vi "Test Worker Registered with Worker Handler after Handling Job.vi"(8 "error in (no error)":errorcluster, 11 "Worker Test in":refnum<class "Worker Test.lvclass">) -> (0 "error out":errorcluster, 3 "Worker Test out":refnum<class "Worker Test.lvclass">)   [LabVIEW 2020, in "Worker Test.lvclass"]
uses:
  Worker Test.lvclass
  C:/Program Files (x86)/National Instruments/LabVIEW 2020/vi.lib/Asteme/LUnit/Test Case.lvclass
  Mock Worker/Mock Job Handler.lvclass
  C:/Users/anton/Documents/GitHub/Triarc-Examples/Coffee Shop/Process Job/Job Handler.lvclass
  <vilib>/Asteme/Triarc Framework/Process/Process.lvclass/Process.ctl
  <vilib>/Asteme/LUnit/Test Case.lvclass/Test Case.ctl
  <vilib>/Asteme/LUnit/LUnit Assertion Result.lvclass/LUnit Assertion Result.ctl
  <vilib>/Asteme/Triarc Framework/Process/Private/SubVIs/Wait for finish.vi
  <vilib>/Asteme/Triarc Framework/Process/Protected/Messaging/Enqueue Message.vi
  <vilib>/Asteme/Triarc Framework/Process/Private/SubVIs/Set Lifecycle State.vi
  <vilib>/Asteme/Triarc Framework/Process/Public/Lifecycle/Get Lifecycle State.vi
  <vilib>/Asteme/LUnit/Palette/Pass If.vi
  <vilib>/Asteme/LUnit/Set Assertion Type.vi
  <vilib>/AdvancedString/1D String Array to Delimited String.vi
  <vilib>/Utility/error.llb/Clear Errors.vi
  <vilib>/Asteme/LUnit/Palette/Fail.vi
  <vilib>/Asteme/LUnit/Palette/Pass.vi
  <vilib>/Asteme/LUnit/LUnit Write Assertion Type.vi
  <vilib>/Asteme/LUnit/Add test result.vi
  <vilib>/Asteme/LUnit/LUnit Write Passed.vi
  <vilib>/Asteme/LUnit/LUnit Get Test Case.vi
  <vilib>/Asteme/LUnit/Assertion Result/LUnit Get Test Name.vi
  <vilib>/Asteme/LUnit/LUnit Write Message.vi
  <vilib>/Asteme/LUnit/LUnit Write Description.vi
  <vilib>/Asteme/LUnit/Read Test Case Name.vi
  Worker/Worker.lvclass
  C:/Program Files (x86)/National Instruments/LabVIEW 2020/vi.lib/Asteme/Triarc Framework/Process/Process.lvclass
  <vilib>/Utility/error.llb/Error Cluster From Error Code.vi
  <vilib>/Asteme/LUnit/LUnit Assertion Result.lvclass
  <vilib>/Asteme/Triarc Framework/Process/Process.lvclass
  <vilib>/Asteme/LUnit/Test Case.lvclass
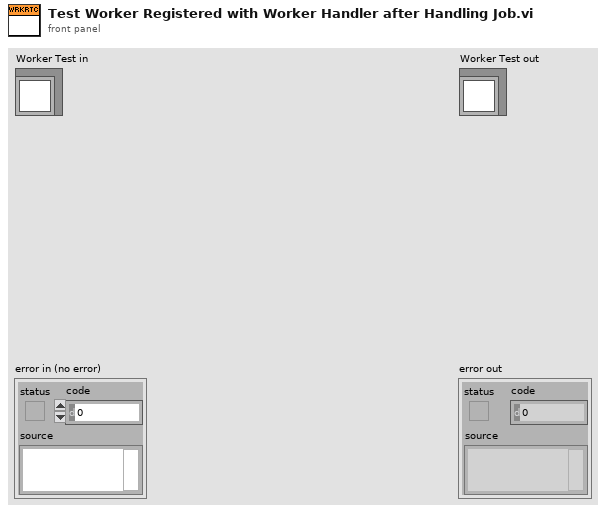
[diagram p1: front panel]
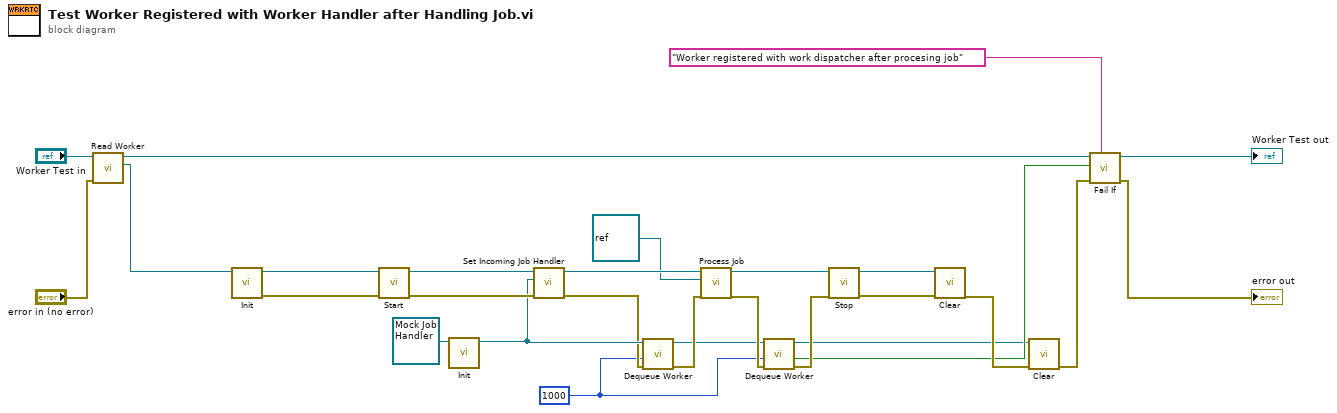
[diagram p0: block diagram]
diagram:
  w1 = 1000 ("timeout in ms (-1)")
  n1 = call "Read Worker.vi"("error in (no error)"="error in (no error)", "Worker Test in"="Worker Test in") -> ("Worker"=w23:refnum<class "Worker.lvclass">, "Worker Test out"=w25:refnum<class "Worker Test.lvclass">)  [unwired: 7 in, 1 out]
  n2 = call-dynamic "Init.vi"("View In"=w23) -> ("error out"=w22:errorcluster, "View Out"=w19:refnum<class "Worker.lvclass">)  [unwired: 9 in]
  n3 = call <vilib>:"Start.vi"("error in (no error)"=w22, "Process In"=w19) -> ("error out"=w18:errorcluster, "Process Out"=w16:refnum<class "Worker.lvclass">)  [unwired: 8 in]
  n4 = call-dynamic "Init.vi"("Mock Job Handler In"=refnum<class "Mock Job Handler.lvclass"> refnum ("Mock Worker In")) -> ("Mock Job Handler Out"=w14:refnum<class "Mock Job Handler.lvclass">)  [unwired: 9 in, 1 out]
  n5 = call "Set Incoming Job Handler.vi"("error in (no error)"=w18, "Job Handler"=w14, "Worker In"=w16) -> ("error out"=w13:errorcluster, "Worker Out"=w9:refnum<class "Worker.lvclass">)  [unwired: 7 in]
  n6 = call "Dequeue Worker.vi"("error in (no error)"=w13, "timeout in ms (-1)"=w1, "Mock Job Handler In"=w14) -> ("error out"=w12:errorcluster, "Mock Job Handler Out"=w3:refnum<class "Mock Job Handler.lvclass">)  [unwired: 5 in, 2 out]
  n7 = call-dynamic "Process Job.vi"("error in (no error)"=w12, "Job"=refnum<class> refnum ("Task"), "Worker In"=w9) -> ("error out"=w6:errorcluster, "Worker Out"=w8:refnum<class "Worker.lvclass">)  [unwired: 7 in]
  n8 = call "Dequeue Worker.vi"("error in (no error)"=w6, "timeout in ms (-1)"=w1, "Mock Job Handler In"=w3) -> ("error out"=w5:errorcluster, "timed out?"=w4:bool, "Mock Job Handler Out"=w2:refnum<class "Mock Job Handler.lvclass">)  [unwired: 5 in, 1 out]
  n9 = call <vilib>:"Stop.vi"("error in (no error)"=w5, "Process In"=w8) -> ("error out"=w20:errorcluster, "Process Out"=w21:refnum<class "Worker.lvclass">)  [unwired: 7 in, 1 out]
  n10 = call-dynamic "Clear.vi"("error in (no error)"=w20, "View In"=w21) -> ("error out"=w11:errorcluster)  [unwired: 9 in]
  n11 = call-dynamic "Clear.vi"("error in (no error)"=w11, "Mock Job Handler In"=w2) -> ("error out"=w10:errorcluster)  [unwired: 9 in]
  n12 = call <vilib>:"Fail If.vi"("Description"="Worker registered with work dispatcher after procesing job", "error in (no error)"=w10, "Fail?"=w4, "Test Case In"=w25) -> ("error out"=→"error out":errorcluster, "Test Case Out"=→"Worker Test out":refnum<class "Worker Test.lvclass">)  [unwired: 6 in]
